vi "calculo_m_H2 (SubVI).vi"(8 "V":dbl, 11 "P":dbl) -> (3 "Numeric out":dbl)   [LabVIEW 2024]
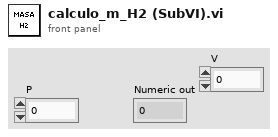
[diagram p1: front panel]
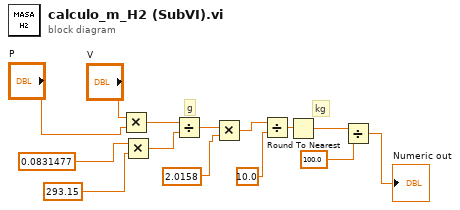
[diagram p0: block diagram]
diagram:
  # "kg"
  # "g"
  n1 = Multiply(x="V", y="P") -> (x*y=w5:dbl)
  n2 = Multiply(x=0.0831477 ("y"), y=293.15) -> (x*y=w3:dbl)
  n3 = Divide(x=w5, y=w3) -> (x/y=w2:dbl)
  n4 = Multiply(x=w2, y=2.0158) -> (x*y=w12:dbl)
  n5 = Divide(x=w12, y=10.0) -> (x/y=w8:dbl)
  n6 = Round To Nearest(number=w8) -> (nearest integer value=w9:dbl)
  n7 = Divide(x=w9, y=100.0) -> (x/y=→"Numeric out":dbl)
